vi "Insert date time into cell.vi"(8 "error in (no error)":errorcluster, 10 "Date/Time Cell":string, 11 "NI_report in":refnum<class "NI_report.lvclass">) -> (0 "error out":errorcluster, 3 "NI_report out":refnum<class "NI_report.lvclass">)   [LabVIEW 2016]
uses:
  <vilib>/Utility/NIReport.llb/NI_report.lvclass
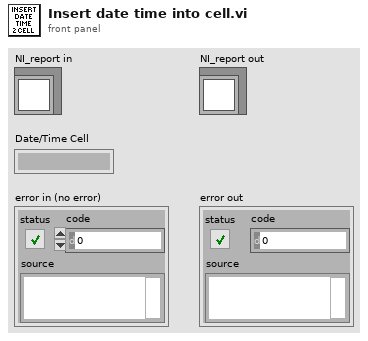
[diagram p1: front panel]
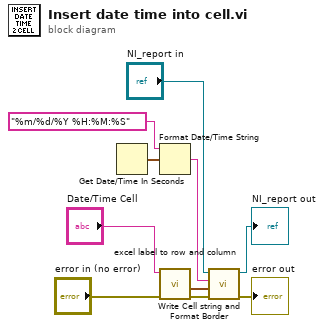
[diagram p0: block diagram]
diagram:
  n1 = Get Date/Time In Seconds() -> (seconds since 1Jan1904=w2:timestamp)
  n2 = Format Date/Time String(time format string (%c)="%m/%d/%Y %H:%M:%S", seconds (now)=w2) -> (date/time string=w8:string)  [unwired: 1 in]
  n3 = call "excel label to row and column.vi"("error in (no error)"="error in (no error)", "cell's name"="Date/Time Cell") -> ("error IO"=w6:errorcluster, "output cluster"=w1:cluster{"row":i32, "column":i32})  [unwired: 5 in, 3 out]
  n4 = call "Write Cell string and Format Border.vi"("error in (no error)"=w6, "output cluster"=w1, "input string"=w8, "NI_report in"="NI_report in") -> ("error out"=→"error out":errorcluster, "NI_report out"=→"NI_report out":refnum<class "NI_report.lvclass">)  [unwired: 6 in]
